vi "Query System Parameters.vi"(8 "error in (no error)":errorcluster, 11 "VISA resource name":refnum<visa-resource-name>) -> (0 "error out":errorcluster, 2 "System Parameters":T1={"Sys Period"=0.1, "Sys Mode"=enum."Normal", "Sys Burst #"=10, "Sys DC On"=10, "Sys DC Off"=10, "Sys State"=TRUE, "Sys Gate"=TRUE, "Sys Trig Edge"=TRUE, "Sys Ext Mode"=enum."Disabled", "Sys Trig Lev"=2.5, "Sys Gate Lev "=2.5, "Sys Gate Mode"=enum."Disabled"} {"Sys Gate Lev" format="%.4p"; "Sys Trig Lev" format="%.4p"; "Sys Period" format="%.6p"}, 3 "VISA resource name out":refnum<visa-resource-name>)   [LabVIEW 2020]
doc: "This VI reads the current configuration of the system timer (To)."
uses:
  System Parameters.ctl
  Berkeley Nucleonics 500 Series.lvlib
panel:
  # "Input"
  # "Triggered"
  # "Gated"
  # "Mode"
  # "Burst"
  # "Duty\nCycle"
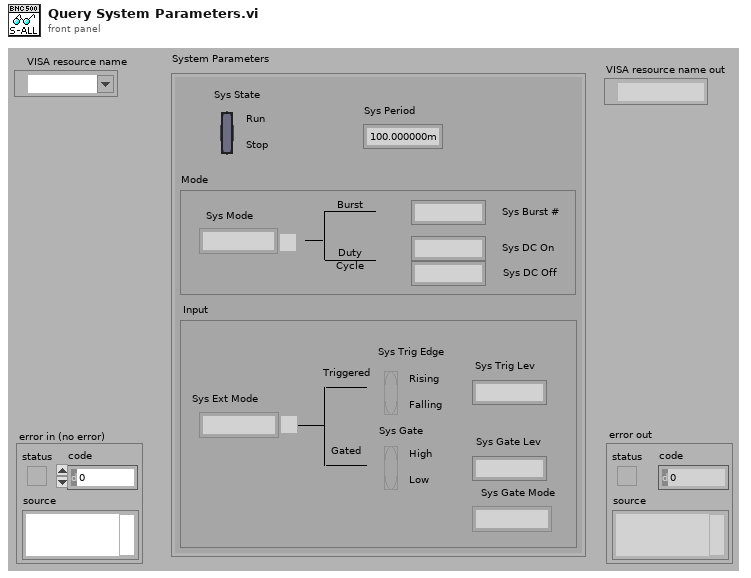
[diagram p1: front panel]
types:
  T1 = typedef "System Parameters.ctl" = cluster{"Sys Period":dbl, "Sys Mode":enum16{"Normal", "Single", "Burst", "Duty Cycle"}, "Sys Burst #":i32, "Sys DC On":i32, "Sys DC Off":i32, "Sys State":bool, "Sys Gate":bool, "Sys Trig Edge":bool, "Sys Ext Mode":enum16{"Disabled", "Triggered", "Gated", "Triggered & Gated"}, "Sys Trig Lev":dbl, "Sys Gate Lev ":dbl, "Sys Gate Mode":enum16{"Disabled", "Pulse Inhibit", "Output Inhibit", "Channel"}}
  T2 = cluster{" Mode":enum16{"Normal", "Single", "Burst", "Duty Cycle"}, "Burst #":i32, "DC Off":i32, "DC On":i32, "Period":dbl}
  T3 = enum16{"Normal", "Single", "Burst", "Duty Cycle"}
  T4 = cluster{"Sys Ext Mode":enum16{"Disabled", "Triggered", "Gated", "Triggered & Gated"}, "Trig Level":dbl, "Trig Edge":bool, "Gate Logic":bool, "Gate Level":dbl, "Gate Mode":enum16{"Disabled", "Pulse Inhibit", "Output Inhibit", "Channel"}}
  T5 = enum16{"Disabled", "Triggered", "Gated", "Triggered & Gated"}
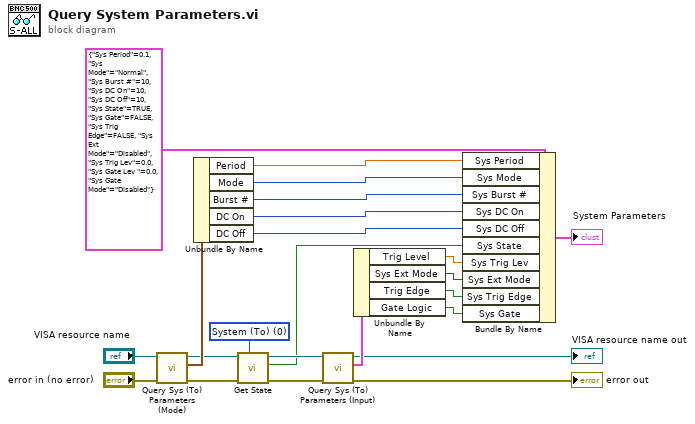
[diagram p0: block diagram]
diagram:
  w23 = 0 items=["System (To)", "Channel A", "Channel B", "Channel C", "Channel D", "Channel E", "Channel F", "Channel G", "Channel H"] ("Channel (1: Chan A)")
  n1 = call "Query Sys (To) Parameters (Mode).vi"("error in (no error)"="error in (no error)", "VISA resource name"="VISA resource name") -> ("error out"=w17:errorcluster, "Mode Parameters"=w22:T2, "VISA resource name out"=w18:refnum<visa-resource-name>)  [unwired: 7 in]
  n2 = Unbundle By Name(w22) -> ("Period"=w11:dbl, "Mode"=w10:T3, "Burst #"=w9:i32, "DC On"=w8:i32, "DC Off"=w7:i32)
  n3 = call "Get State.vi"("Channel (1: Chan A)"=w23, "error in (no error)"=w17, "VISA resource name"=w18) -> ("error out"=w15:errorcluster, "State"=w6:bool, "VISA resource name out"=w16:refnum<visa-resource-name>)  [unwired: 6 in]
  n4 = call "Query Sys (To) Parameters (Input).vi"("error in (no error)"=w15, "VISA resource name"=w16) -> ("error out"=→"error out":errorcluster, "Input Parameters"=w21:T4, "VISA resource name out"=→"VISA resource name out":refnum<visa-resource-name>)  [unwired: 7 in]
  n5 = Unbundle By Name(w21) -> ("Trig Level"=w5:dbl, "Sys Ext Mode"=w4:T5, "Trig Edge"=w3:bool, "Gate Logic"=w2:bool)
  n6 = Bundle By Name(cluster=T1 {"Sys Period"=0.1, "Sys Mode"=enum."Normal", "Sys Burst #"=10, "Sys DC On"=10, "Sys DC Off"=10, "Sys State"=TRUE, "Sys Gate"=FALSE, "Sys Trig Edge"=FALSE, "Sys Ext Mode"=enum."Disabled", "Sys Trig Lev"=0.0, "Sys Gate Lev "=0.0, "Sys Gate Mode"=enum."Disabled"} ("System Parameters"), "Sys Period"=w11, "Sys Mode"=w10, "Sys Burst #"=w9, "Sys DC On"=w8, "Sys DC Off"=w7, "Sys State"=w6, "Sys Trig Lev"=w5, "Sys Ext Mode"=w4, "Sys Trig Edge"=w3, "Sys Gate"=w2) -> (→"System Parameters":T1)
